vi "Increment Build Number.vi"(0 "Compound_Installer in":refnum<class "Compound_Installer.lvclass">, 11 "error in (no error)":errorcluster) -> (4 "Compound_Installer out":refnum<class "Compound_Installer.lvclass">, 15 "error out":errorcluster)   [LabVIEW 2017, in "CL_G3_VIComponentBuilder.lvlib" / "Compound_Installer.lvclass"]
doc: "The must override from the parent. This function has no implementation."
uses:
  Compound_Installer.lvclass
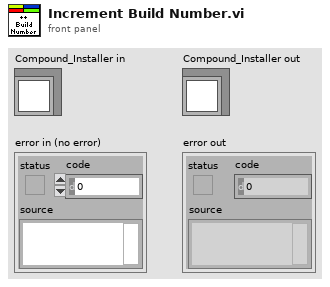
[diagram p1: front panel]
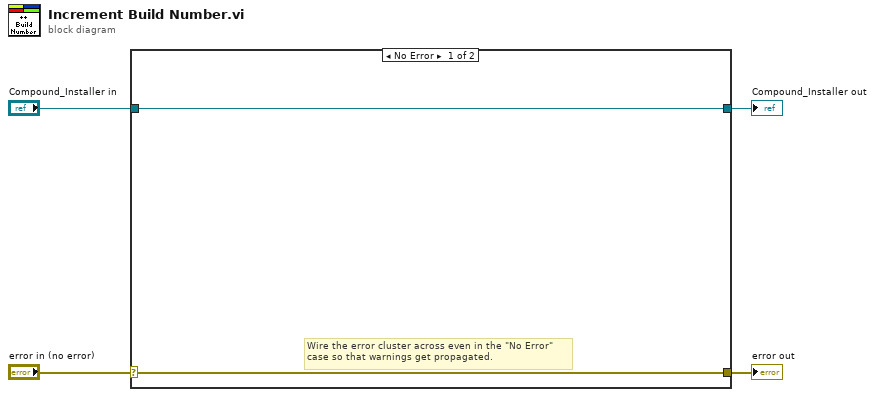
[diagram p0: block diagram]
diagram:
  n1 = case shown="No Error" "error in (no error)" {
    selector: "error in (no error)" -> [w5 w8]
    tunnel: [w5 w8] -> w3
    tunnel: [w6 w7] -> w1
    tunnel: "Compound_Installer in" -> [w6 w7]
    frame No Error {
      # "Wire the error cluster across even in the \"No Error\"\ncase so that warnings get propagated."
    }
    frame Error {
    }
  }
  "error out" <- w3
  "Compound_Installer out" <- w1
